vi "映射距离矩阵.vi"(0 "距离":dbl=1.0 format="%#_13g") -> (14 "平移采样点信息":dbl[][](array[numeric]))   [LabVIEW 2018]
uses:
  <vilib>/Utility/file.llb/Read Delimited Spreadsheet (DBL).vi
panel:
  out "阵列坐标":dbl[][](array[numeric])
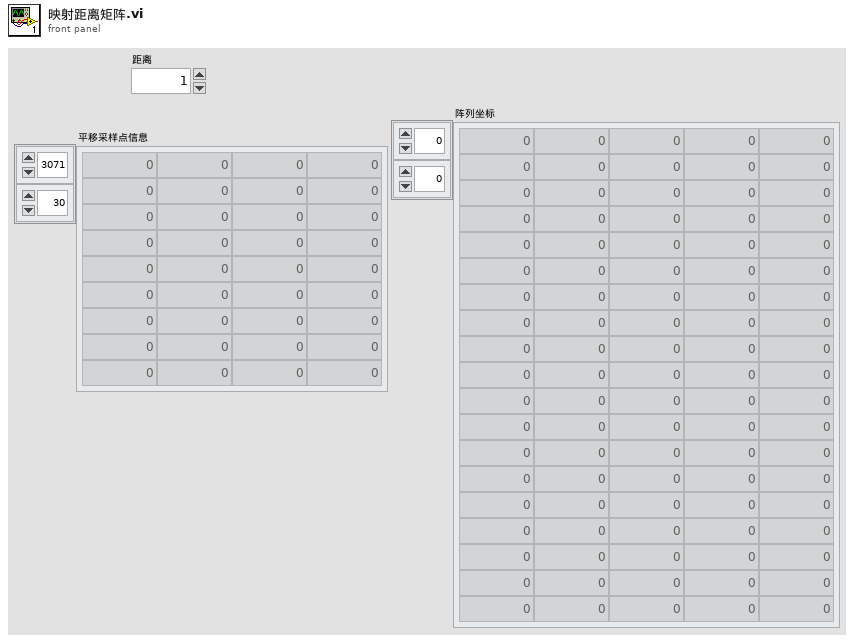
[diagram p1: front panel]
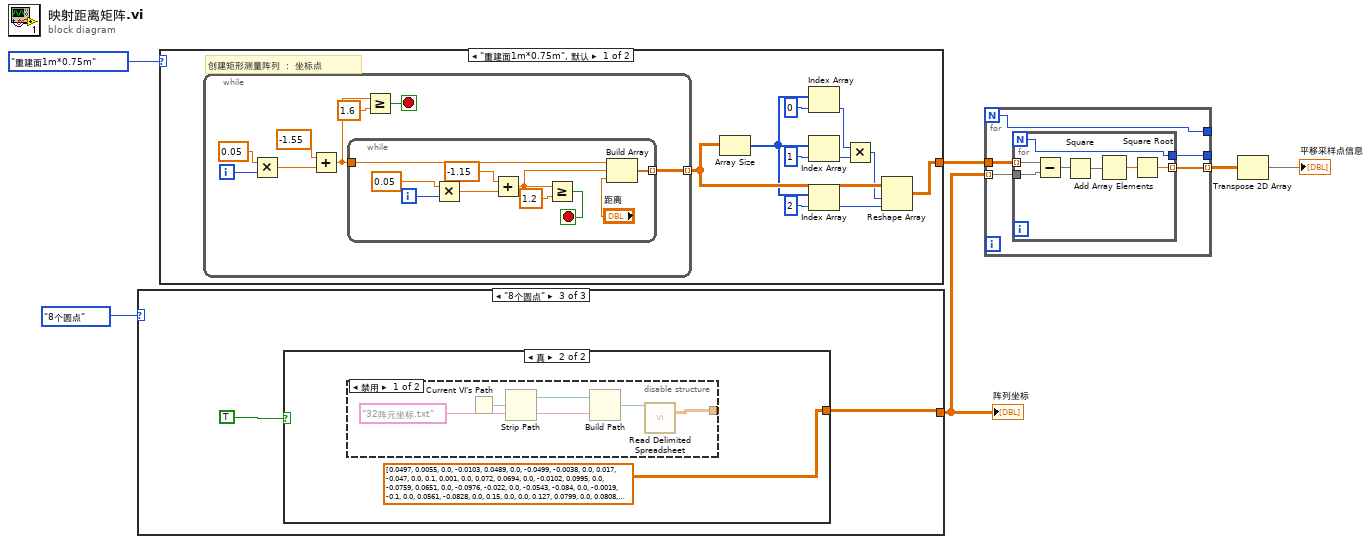
[diagram p0: block diagram]
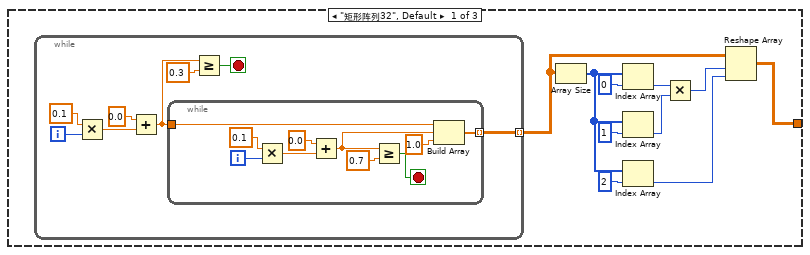
[diagram p2: hidden frame]
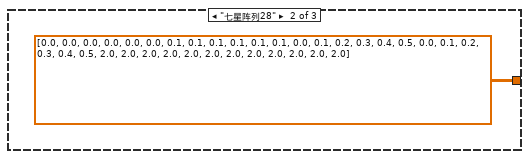
[diagram p3: hidden frame]
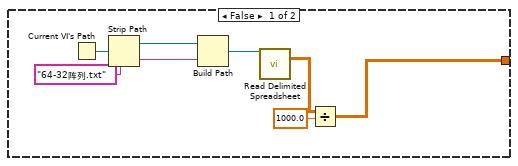
[diagram p4: hidden frame]
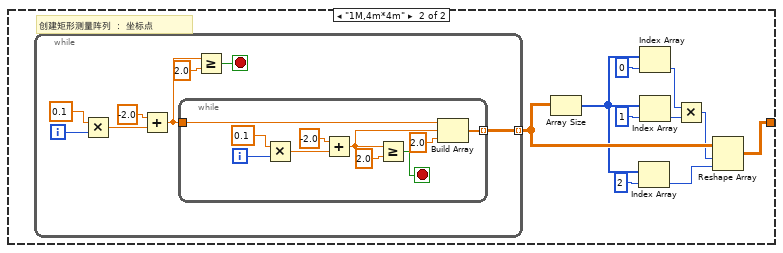
[diagram p6: hidden frame]
diagram:
  n1 = case shown="\"8个圆点\"" enum16{"矩形阵列32", "8个圆点", "七星阵列28", ""}."8个圆点" ("操作(0:open)") {
    tunnel: [w7 dbl[][] [[0.0, 0.0, 0.0, 0.0, 0.0, 0.0, 0.1, 0.1, 0.1, 0.1, 0.1, 0.1], [0.0, 0.1, 0.2, 0.3, 0.4, 0.5, 0.0, 0.1, 0.2, 0.3, 0.4, 0.5], [2.0, 2.0, 2.0, 2.0, 2.0, 2.0, 2.0, 2.0, 2.0, 2.0, 2.0, 2.0]] w37] -> w3
    frame "矩形阵列32", Default {
      n2 = while {
        tunnel: [w17] -> w8 mode=indexing
        i -> [w24]
        stop <- w20 stop-if-true
        n3 = Multiply(x=0.1, y=w24) -> (x*y=w22:dbl)
        n4 = Add(x=0.0, y=w22) -> (x+y=w18:dbl)
        n5 = while {
          tunnel: [w26] -> w17 mode=indexing
          tunnel: w18 -> [w28]
          i -> [w29]
          stop <- w31 stop-if-true
          n6 = Multiply(x=0.1, y=w29) -> (x*y=w33:dbl)
          n7 = Add(x=0.0, y=w33) -> (x+y=w27:dbl)
          n8 = Greater Or Equal?(x=w27, y=0.7) -> (x >= y?=w31:bool)
          n9 = Build Array(w28, w27, 1.0 ("元素")) -> (w26:dbl[])
        }
        n10 = Greater Or Equal?(x=w18, y=0.3) -> (x >= y?=w20:bool)
      }
      n11 = Array Size(array=w8) -> (size(s)=w13:i32[])
      n12 = Index Array(array=w13, index=0 ("索引")) -> (element=w12:i32)
      n13 = Index Array(array=w13, index=1 ("索引")) -> (element=w11:i32)
      n14 = Index Array(array=w13, index=2 ("索引")) -> (element=w9:i32)
      n15 = Multiply(x=w12, y=w11) -> (x*y=w10:i32)
      n16 = Reshape Array(w8, w10, w9) -> (w7:dbl[][])
    }
    frame "七星阵列28" {
    }
    frame "8个圆点" {
      n17 = case shown="真" TRUE {
        tunnel: [w40 dbl[][] [[0.0497, 0.0055, 0.0], [-0.0103, 0.0489, 0.0], [-0.0499, -0.0038, 0.0], [0.017, -0.047, 0.0], [0.1, 0.001, 0.0], [0.072, 0.0694, 0.0], [-0.0102, 0.0995, 0.0], [-0.0759, 0.0651, 0.0], [-0.0976, -0.022, 0.0], [-0.0543, -0.084, 0.0], [-0.0019, -0.1, 0.0], [0.0561, -0.0828, 0.0], [0.15, 0.0, 0.0], [0.127, 0.0799, 0.0], [0.0808, 0.1263, 0.0], [-0.0037, 0.15, 0.0], [-0.0612, 0.137, 0.0], [-0.1195, 0.0907, 0.0], [-0.1499, -0.0039, 0.0], [-0.1329, -0.0696, 0.0], [-0.0859, -0.123, 0.0], [-0.0192, -0.1488, 0.0], [0.0741, -0.1304, 0.0], [0.1346, -0.0661, 0.0], [0.2, -0.0034, 0.0], [0.1901, 0.0622, 0.0], [0.1521, 0.1299, 0.0], [0.0744, 0.1857, 0.0], [0.014, 0.1995, 0.0], [-0.0681, 0.1881, 0.0], [-0.1485, 0.1339, 0.0], [-0.1917, 0.057, 0.0]] ("all rows")] -> w37
        frame False {
          n18 = Current VI's Path() -> (path=w42:path)
          n19 = Strip Path(path=w42) -> (stripped path=w38:path)  [unwired: 1 out]
          n20 = Build Path(base path=w38, name or relative path="64-32阵列.txt" ("名称或相对路径")) -> (appended path=w43:path)
          n21 = call-poly <vilib>:"Read Delimited Spreadsheet.vi"("file path (dialog if empty)"=w43) -> ("all rows"=w41:dbl[][])  [unwired: 9 in, 5 out]
          n22 = Divide(x=w41, y=1000.0) -> (x/y=w40:dbl[][])
        }
        frame True {
          n23 = disable-structure shown="禁用" {
            disable-tunnel: [w47 _] -> _
            frame Disabled {
              n24 = Current VI's Path() -> (path=w49:path)
              n25 = Strip Path(path=w49) -> (stripped path=w48:path)  [unwired: 1 out]
              n26 = Build Path(base path=w48, name or relative path="32阵元坐标.txt" ("名称或相对路径")) -> (appended path=w50:path)
              n27 = call-poly <vilib>:"Read Delimited Spreadsheet.vi"("file path (dialog if empty)"=w50) -> ("all rows"=w47:dbl[][])  [unwired: 9 in, 5 out]
            }
            frame Enabled {
            }
          }
        }
      }
    }
  }
  "阵列坐标" <- w3
  n28 = case shown="\"重建面1m*0.75m\", 默认" enum16{"重建面1m*0.75m", "1M,4m*4m", ""}."重建面1m*0.75m" ("操作(0:open)") {
    tunnel: [w51 w79] -> w5
    frame "重建面1m*0.75m", Default {
      # "创建矩形测量阵列 ： 坐标点"
      n29 = while {
        tunnel: [w61] -> w60 mode=indexing
        i -> [w68]
        stop <- w64 stop-if-true
        n30 = Multiply(x=0.05, y=w68) -> (x*y=w66:dbl)
        n31 = Add(x=-1.55, y=w66) -> (x+y=w62:dbl)
        n32 = while {
          tunnel: [w70] -> w61 mode=indexing
          tunnel: w62 -> [w72]
          i -> [w73]
          stop <- w75 stop-if-true
          n33 = Multiply(x=0.05, y=w73) -> (x*y=w77:dbl)
          n34 = Add(x=-1.15, y=w77) -> (x+y=w71:dbl)
          n35 = Greater Or Equal?(x=w71, y=1.2) -> (x >= y?=w75:bool)
          n36 = Build Array(w72, w71, "距离") -> (w70:dbl[])
        }
        n37 = Greater Or Equal?(x=w62, y=1.6) -> (x >= y?=w64:bool)
      }
      n38 = Array Size(array=w60) -> (size(s)=w56:i32[])
      n39 = Index Array(array=w56, index=0 ("索引")) -> (element=w55:i32)
      n40 = Index Array(array=w56, index=1 ("索引")) -> (element=w54:i32)
      n41 = Index Array(array=w56, index=2 ("索引")) -> (element=w52:i32)
      n42 = Multiply(x=w55, y=w54) -> (x*y=w53:i32)
      n43 = Reshape Array(w60, w53, w52) -> (w51:dbl[][])
    }
    frame "1M,4m*4m" {
      # "创建矩形测量阵列 ： 坐标点"
      n44 = while {
        tunnel: [w89] -> w88 mode=indexing
        i -> [w96]
        stop <- w92 stop-if-true
        n45 = Multiply(x=0.1, y=w96) -> (x*y=w94:dbl)
        n46 = Add(x=-2.0, y=w94) -> (x+y=w90:dbl)
        n47 = while {
          tunnel: [w98] -> w89 mode=indexing
          tunnel: w90 -> [w100]
          i -> [w101]
          stop <- w103 stop-if-true
          n48 = Multiply(x=0.1, y=w101) -> (x*y=w105:dbl)
          n49 = Add(x=-2.0, y=w105) -> (x+y=w99:dbl)
          n50 = Greater Or Equal?(x=w99, y=2.0) -> (x >= y?=w103:bool)
          n51 = Build Array(w100, w99, 2.0) -> (w98:dbl[])
        }
        n52 = Greater Or Equal?(x=w90, y=2.0) -> (x >= y?=w92:bool)
      }
      n53 = Array Size(array=w88) -> (size(s)=w84:i32[])
      n54 = Index Array(array=w84, index=2 ("索引")) -> (element=w80:i32)
      n55 = Index Array(array=w84, index=0 ("索引")) -> (element=w83:i32)
      n56 = Index Array(array=w84, index=1 ("索引")) -> (element=w82:i32)
      n57 = Multiply(x=w83, y=w82) -> (x*y=w81:i32)
      n58 = Reshape Array(w88, w81, w80) -> (w79:dbl[][])
    }
  }
  n59 = for {
    N -> [w107]
    tunnel: w3 -> [w111] mode=indexing
    tunnel: w5 -> [w110]
    tunnel: [w109] -> w4 mode=indexing
    tunnel: [w108] -> _
    tunnel: [w107] -> _
    n60 = for {
      N -> [w112]
      tunnel: w111 -> [w117]
      tunnel: w110 -> [w118] mode=indexing
      tunnel: [w113] -> w109 mode=indexing
      tunnel: [w112] -> w108
      n61 = Subtract(x=w118, y=w117) -> (x-y=w116:dbl[])
      n62 = Square(x=w116) -> (x^2=w115:dbl[])
      n63 = Add Array Elements(numeric array=w115) -> (sum=w114:dbl)
      n64 = Square Root(x=w114) -> (sqrt(x)=w113:dbl)
    }
  }
  n65 = Transpose 2D Array(2D array=w4) -> (transposed array=→"平移采样点信息":dbl[][])
